vi "file -- scan filename logic -- V1.vi"(7 "scan fileneme action":T1, 8 "scan filename IN":T2={"mmddyy (str)"="", "counter (str)"="", "to F (kHz)"=0.0, "from F (kHz)"=0.0, "temperature (K)"=0.0, "date/time string"="", "time stamp"=timestamp(19856294.882018566 s since 1904-01-01), "base name"="", "temperature (str)"="", "from F (str)"="", "to F (str)"="", "format"=enum."no date string", "power (V)"=0.0, "power (str) "="", "Magn Field (T)"=0.0, "Magn Field (str)"=""}, 11 "base name IN":string="1.02000K_12_177_1.4V_Nov09-2012__12-14-10_001_110912") -> (0 "scan filename OUT":T2={"mmddyy (str)"="", "counter (str)"="", "to F (kHz)"=0.0, "from F (kHz)"=0.0, "temperature (K)"=0.0, "date/time string"="", "time stamp"=timestamp(19856294.882018566 s since 1904-01-01), "base name"="", "temperature (str)"="", "from F (str)"="", "to F (str)"="", "format"=enum."no date string", "power (V)"=0.0, "power (str) "="", "Magn Field (T)"=0.0, "Magn Field (str)"=""}, 1 "exact match":bool, 3 "string OUT":string)   [LabVIEW 2016]
uses:
  resonant_ultrasound/maglab ultrasound -- arkady/file -- scan filename.ctl
  resonant_ultrasound/maglab ultrasound -- arkady/file -- scan filename action.ctl
  <vilib>/regexp/Match Regular Expression.xnode
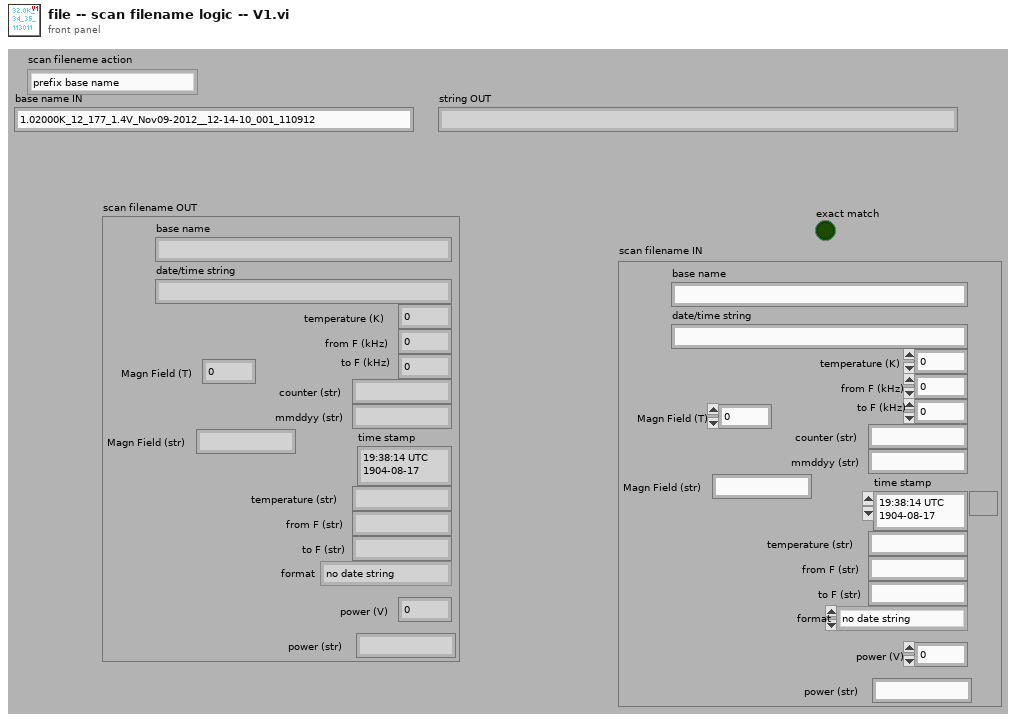
[diagram p1: front panel]
types:
  T1 = typedef "file -- scan filename action.ctl" = enum16{"prefix base name", "datestring regexp", "parse datestring", "datestring", "filename regexp", "parse filename", "datestring regexp (no brackets)", "suffix base name"}
  T2 = typedef "file -- scan filename.ctl" = cluster{"mmddyy (str)":string, "counter (str)":string, "to F (kHz)":dbl, "from F (kHz)":dbl, "temperature (K)":dbl, "date/time string":string, "time stamp":timestamp, "base name":string, "temperature (str)":string, "from F (str)":string, "to F (str)":string, "format":enum16{"no date string", "with date string"}, "power (V)":dbl, "power (str) ":string, "Magn Field (T)":dbl, "Magn Field (str)":string}
  T3 = typedef "LVDateTimeRec.ctl" = cluster{"fractional second":dbl, "second":i32, "minute":i32, "hour":i32, "day of month":i32, "month":i32, "year":i32, "day of week":i32, "day of year":i32, "DST":i32}
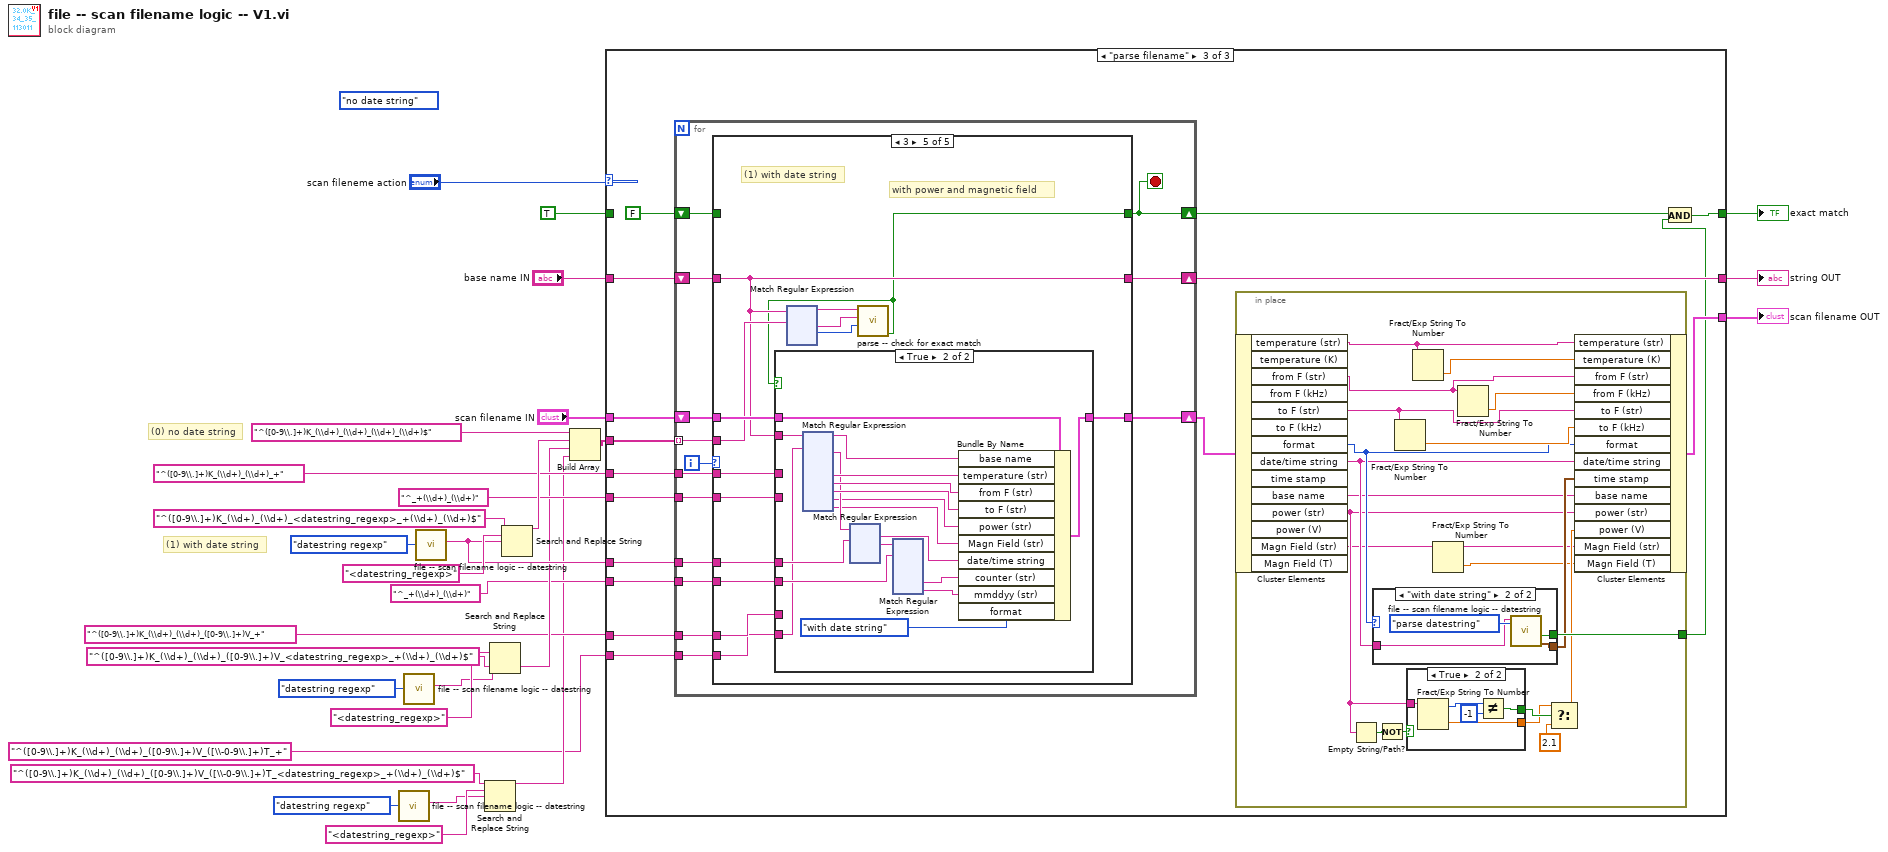
[diagram p0: block diagram]
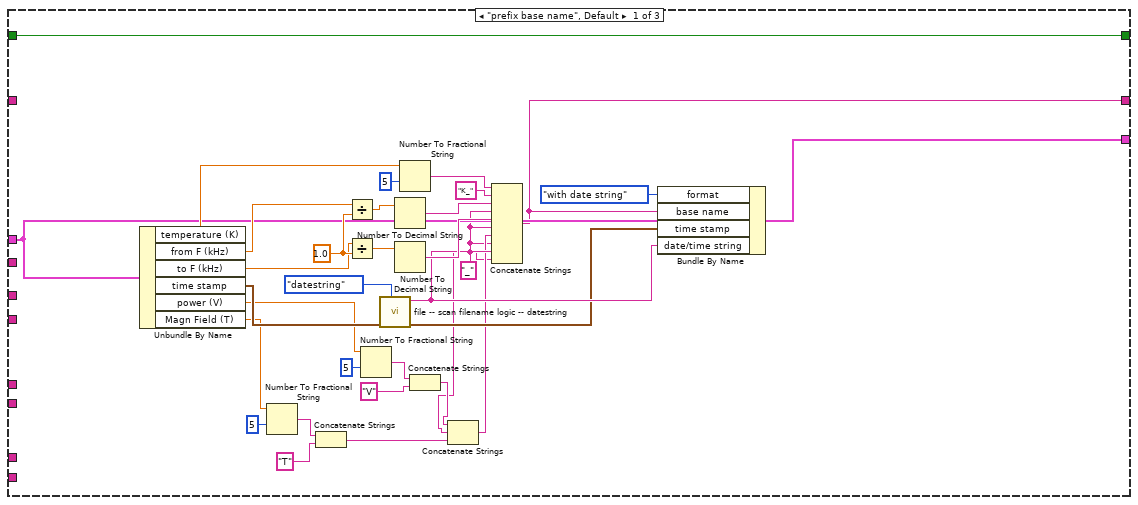
[diagram p2: hidden frame]
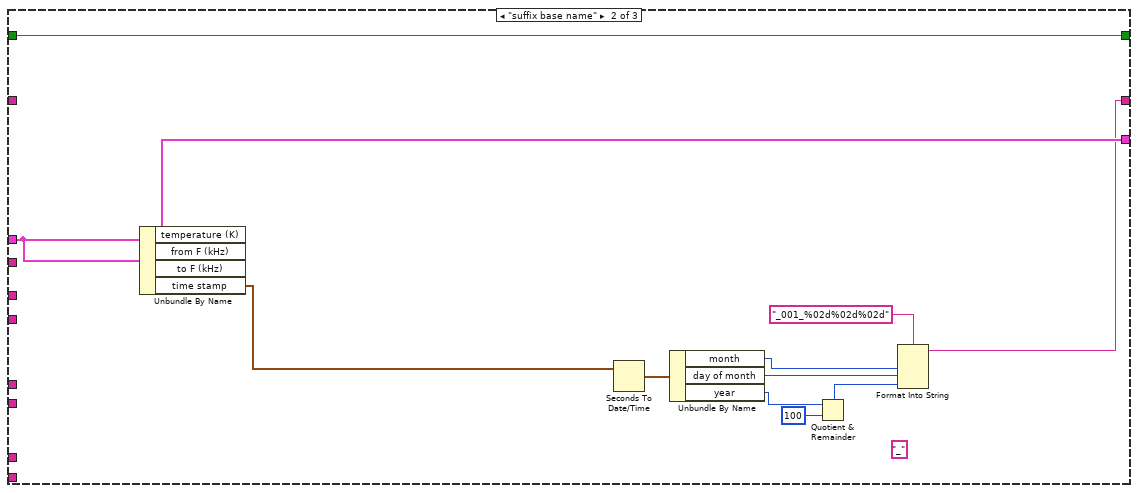
[diagram p3: hidden frame]
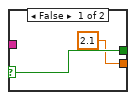
[diagram p4: hidden frame]
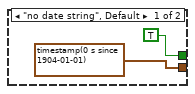
[diagram p5: hidden frame]
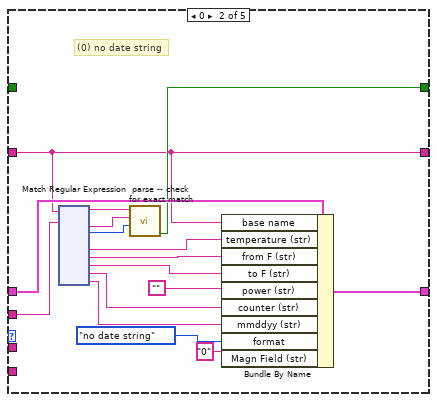
[diagram p7: hidden frame]
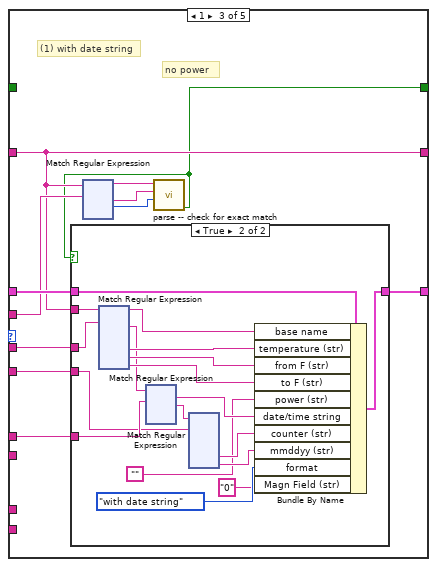
[diagram p8: hidden frame]
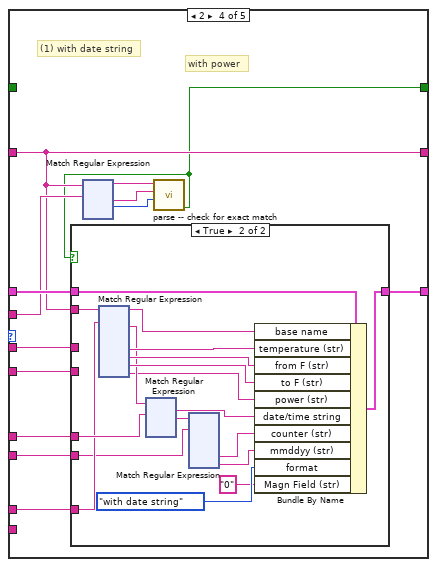
[diagram p10: hidden frame]
diagram:
  (unwired) enum16{"no date string", "with date string"}."no date string"
  # "(1) with date string"
  # "(0) no date string"
  n1 = call "file -- scan filename logic -- datestring.vi"("scan filename action"=file_--_scan_filename_action."datestring regexp") -> ("date string regexp"=w4:string)  [unwired: 7 in, 3 out]
  n2 = call "file -- scan filename logic -- datestring.vi"("scan filename action"=file_--_scan_filename_action."datestring regexp") -> ("date string regexp"=w11:string)  [unwired: 7 in, 3 out]
  n3 = call "file -- scan filename logic -- datestring.vi"("scan filename action"=file_--_scan_filename_action."datestring regexp") -> ("date string regexp"=w15:string)  [unwired: 7 in, 3 out]
  n4 = Search and Replace String(input string="^([0-9\\.]+)K_(\\d+)_(\\d+)_([0-9\\.]+)V_([\\-0-9\\.]+)T_<datestring_regexp>_+(\\d+)_(\\d+)$" ("string"), search string="<datestring_regexp>" ("string"), replace string=w4) -> (result string=w2:string)  [unwired: 5 in, 3 out]
  n5 = Search and Replace String(input string="^([0-9\\.]+)K_(\\d+)_(\\d+)_([0-9\\.]+)V_<datestring_regexp>_+(\\d+)_(\\d+)$" ("string"), search string="<datestring_regexp>" ("string"), replace string=w11) -> (result string=w9:string)  [unwired: 5 in, 3 out]
  n6 = Search and Replace String(input string="^([0-9\\.]+)K_(\\d+)_(\\d+)_<datestring_regexp>_+(\\d+)_(\\d+)$" ("string"), search string="<datestring_regexp>" ("string"), replace string=w15) -> (result string=w19:string)  [unwired: 5 in, 3 out]
  n7 = Build Array("^([0-9\\.]+)K_(\\d+)_(\\d+)_(\\d+)_(\\d+)$" ("string"), w19, w9, w2) -> (w18:string[])
  n8 = case shown="\"parse filename\"" "scan fileneme action" {
    tunnel: [w48 w72 w80] -> w29
    tunnel: "base name IN" -> [_ _ w84]
    tunnel: [w46 w67 w82] -> w17
    tunnel: "scan filename IN" -> [w47 w67 w88]
    tunnel: [w43 w62 w85] -> w25
    tunnel: TRUE -> [w48 w72 _]
    tunnel: w18 -> [_ _ w86]
    tunnel: "^([0-9\\.]+)K_(\\d+)_(\\d+)_+" ("string") -> [_ _ w78]
    tunnel: w15 -> [_ _ w77]
    tunnel: "^_+(\\d+)_(\\d+)" ("string") -> [_ _ w76]
    tunnel: "^([0-9\\.]+)K_(\\d+)_(\\d+)_([0-9\\.]+)V_+" ("string") -> [_ _ w75]
    tunnel: "^_+(\\d+)_(\\d+)" ("string") -> [_ _ w74]
    tunnel: "^([0-9\\.]+)K_(\\d+)_(\\d+)_([0-9\\.]+)V_([\\-0-9\\.]+)T_+" ("string") -> [_ _ w73]
    frame "prefix base name", Default {
      w57 = 1.0 ("y")
      w31 = "_" ("string")
      n9 = Unbundle By Name(w47) -> ("temperature (K)"=w50:dbl, "from F (kHz)"=w55:dbl, "to F (kHz)"=w56:dbl, "time stamp"=w49:timestamp, "power (V)"=w40:dbl, "Magn Field (T)"=w34:dbl)
      n10 = Number To Fractional String(number=w34, precision (6)=i16 5 ("width (-)")) -> (F-format string=w36:string)  [unwired: 2 in]
      n11 = Concatenate Strings(w36, "T" ("string")) -> (w30:string)
      n12 = Divide(x=w55, y=w57) -> (x/y=w60:dbl)
      n13 = Divide(x=w56, y=w57) -> (x/y=w59:dbl)
      n14 = Number To Fractional String(number=w40, precision (6)=i16 5 ("width (-)")) -> (F-format string=w39:string)  [unwired: 2 in]
      n15 = call "file -- scan filename logic -- datestring.vi"("scan filename action"=file_--_scan_filename_action."datestring", "time stamp IN"=w49) -> ("time stamp OUT"=w44:timestamp, "date/time string OUT"=w45:string)  [unwired: 6 in, 2 out]
      n16 = Number To Decimal String(number=w60) -> (decimal integer string=w51:string)  [unwired: 1 in]
      n17 = Number To Decimal String(number=w59) -> (decimal integer string=w52:string)  [unwired: 1 in]
      n18 = Number To Fractional String(number=w50, precision (6)=i16 5 ("width (-)")) -> (F-format string=w58:string)  [unwired: 2 in]
      n19 = Concatenate Strings(w39, "V" ("string")) -> (w33:string)
      n20 = Concatenate Strings(w33, w31, w30) -> (w32:string)
      n21 = Concatenate Strings(w58, "K_" ("string"), w51, w31, w52, w31, w32, w31, w45, w31) -> (w43:string)
      n22 = Bundle By Name(cluster=w47, "format"=enum16{"no date string", "with date string"}."with date string", "base name"=w43, "time stamp"=w44, "date/time string"=w45) -> (w46:T2)
    }
    frame "suffix base name" {
      (unwired) "_" ("string")
      n23 = Unbundle By Name(w67) -> ("time stamp"=w71:timestamp)  [unwired: 3 out]
      n24 = Seconds To Date/Time(time stamp (now)=w71) -> (date time rec=w70:T3)  [unwired: 1 in]
      n25 = Unbundle By Name(w70) -> ("month"=w66:i32, "day of month"=w65:i32, "year"=w69:i32)
      n26 = Quotient & Remainder(x=w69, y=100) -> (x-y*floor(x/y)=w64:i32)  [unwired: 1 out]
      n27 = Format Into String(format string="_001_%02d%02d%02d", w66, w65, w64) -> (resulting string=w62:string)  [unwired: 2 in, 1 out]
    }
    frame "parse filename" {
      n28 = for {
        shift-right: [w130] -> w81
        shift-left: FALSE -> [w128]
        tunnel: w86 -> [w133] mode=indexing
        shift-right: [w132] -> w85
        shift-left: w84 -> [w131]
        shift-right: [w129] -> w83
        shift-left: w88 -> [w135]
        tunnel: w78 -> [w127]
        tunnel: w77 -> [w126]
        tunnel: w76 -> [w125]
        tunnel: w75 -> [w124]
        tunnel: w74 -> [w123]
        tunnel: w73 -> [w122]
        i -> [w134]
        stop <- w130 stop-if-true
        n29 = case shown="3" w134 {
          tunnel: [w136 w153 w282 w764 w1248] -> w129
          tunnel: w135 -> [w136 w152 w281 w763 w1247]
          tunnel: w131 -> [w138 w146 w276 w758 w1242]
          tunnel: [w137 w148 w275 w757 w1241] -> w130
          tunnel: w133 -> [_ w147 w277 w759 w1243]
          tunnel: [w138 w146 w276 w758 w1242] -> w132
          tunnel: w128 -> [w137 _ _ _ _]
          tunnel: w127 -> [_ _ w274 w756 w1240]
          tunnel: w126 -> [_ _ w273 w755 w1239]
          tunnel: w125 -> [_ _ w272 w754 w1238]
          tunnel: w124 -> [_ _ _ w753 w1237]
          tunnel: w123 -> [_ _ _ w752 w1236]
          tunnel: w122 -> [_ _ _ _ w1235]
          frame -1, Default {
          }
          frame 0 {
            # "(0) no date string"
            n30 = xnode "Match Regular Expression"("input string"=w146, "regular expression"=w147) -> ("before match"=w151:string, "after match"=w150:string, "offset past match"=w149:i32, "submatch 1"=w142:string, "submatch 2"=w143:string, "submatch 3"=w144:string, "submatch 4"=w154:string, "submatch 5"=w145:string)  [unwired: 4 in, 2 out]
            n31 = call "parse -- check for exact match.vi"("offset past match"=w149, "after match"=w150, "before match"=w151) -> ("exact match"=w148:bool)  [unwired: 8 in]
            n32 = Bundle By Name(cluster=w152, "base name"=w146, "temperature (str)"=w142, "from F (str)"=w143, "to F (str)"=w144, "power (str)"="", "counter (str)"=w154, "mmddyy (str)"=w145, "format"=enum16{"no date string", "with date string"}."no date string", "Magn Field (str)"="0") -> (w153:T2)
          }
          frame 1 {
            # "no power"
            # "(1) with date string"
            n33 = xnode "Match Regular Expression"("input string"=w276, "regular expression"=w277) -> ("before match"=w280:string, "after match"=w279:string, "offset past match"=w278:i32)  [unwired: 4 in, 2 out]
            n34 = call "parse -- check for exact match.vi"("offset past match"=w278, "after match"=w279, "before match"=w280) -> ("exact match"=w275:bool)  [unwired: 8 in]
            n35 = case shown="True" w275 {
              tunnel: [w283 w300] -> w282
              tunnel: w281 -> [w283 w299]
              tunnel: w276 -> [_ w298]
              tunnel: w274 -> [_ w297]
              tunnel: w273 -> [_ w292]
              tunnel: w272 -> [_ w289]
              frame False {
              }
              frame True {
                n36 = xnode "Match Regular Expression"("input string"=w298, "regular expression"=w297) -> ("after match"=w293:string, "submatch 1"=w296:string, "submatch 2"=w295:string, "submatch 3"=w294:string)  [unwired: 4 in, 4 out]
                n37 = xnode "Match Regular Expression"("input string"=w293, "regular expression"=w292) -> ("whole match"=w291:string, "after match"=w290:string)  [unwired: 4 in, 3 out]
                n38 = xnode "Match Regular Expression"("input string"=w290, "regular expression"=w289) -> ("submatch 1"=w288:string, "submatch 2"=w287:string)  [unwired: 4 in, 5 out]
                n39 = Bundle By Name(cluster=w299, "base name"=w298, "temperature (str)"=w296, "from F (str)"=w295, "to F (str)"=w294, "power (str)"="", "date/time string"=w291, "counter (str)"=w288, "mmddyy (str)"=w287, "format"=enum16{"no date string", "with date string"}."with date string", "Magn Field (str)"="0") -> (w300:T2)
              }
            }
          }
          frame 2 {
            # "with power"
            # "(1) with date string"
            n40 = xnode "Match Regular Expression"("input string"=w758, "regular expression"=w759) -> ("before match"=w762:string, "after match"=w761:string, "offset past match"=w760:i32)  [unwired: 4 in, 2 out]
            n41 = call "parse -- check for exact match.vi"("offset past match"=w760, "after match"=w761, "before match"=w762) -> ("exact match"=w757:bool)  [unwired: 8 in]
            n42 = case shown="True" w757 {
              tunnel: [w765 w782] -> w764
              tunnel: w763 -> [w765 w781]
              tunnel: w758 -> [_ w780]
              tunnel: w756 -> [_ _]
              tunnel: w755 -> [_ w775]
              tunnel: w754 -> [_ _]
              tunnel: w753 -> [_ w768]
              tunnel: w752 -> [_ w767]
              frame False {
              }
              frame True {
                n43 = xnode "Match Regular Expression"("input string"=w780, "regular expression"=w768) -> ("after match"=w776:string, "submatch 1"=w779:string, "submatch 2"=w778:string, "submatch 3"=w777:string, "submatch 4"=w769:string)  [unwired: 4 in, 4 out]
                n44 = xnode "Match Regular Expression"("input string"=w776, "regular expression"=w775) -> ("whole match"=w774:string, "after match"=w773:string)  [unwired: 4 in, 3 out]
                n45 = xnode "Match Regular Expression"("input string"=w773, "regular expression"=w767) -> ("submatch 1"=w772:string, "submatch 2"=w771:string)  [unwired: 4 in, 5 out]
                n46 = Bundle By Name(cluster=w781, "base name"=w780, "temperature (str)"=w779, "from F (str)"=w778, "to F (str)"=w777, "power (str)"=w769, "date/time string"=w774, "counter (str)"=w772, "mmddyy (str)"=w771, "format"=enum16{"no date string", "with date string"}."with date string", "Magn Field (str)"="0") -> (w782:T2)
              }
            }
          }
          frame 3 {
            # "with power and magnetic field"
            # "(1) with date string"
            n47 = xnode "Match Regular Expression"("input string"=w1242, "regular expression"=w1243) -> ("before match"=w1246:string, "after match"=w1245:string, "offset past match"=w1244:i32)  [unwired: 4 in, 2 out]
            n48 = call "parse -- check for exact match.vi"("offset past match"=w1244, "after match"=w1245, "before match"=w1246) -> ("exact match"=w1241:bool)  [unwired: 8 in]
            n49 = case shown="True" w1241 {
              tunnel: [w1249 w1266] -> w1248
              tunnel: w1247 -> [w1249 w1265]
              tunnel: w1242 -> [_ w1264]
              tunnel: w1240 -> [_ _]
              tunnel: w1239 -> [_ w1259]
              tunnel: w1238 -> [_ _]
              tunnel: w1237 -> [_ _]
              tunnel: w1236 -> [_ w1252]
              tunnel: w1235 -> [_ w1251]
              frame False {
              }
              frame True {
                n50 = xnode "Match Regular Expression"("input string"=w1264, "regular expression"=w1251) -> ("after match"=w1260:string, "submatch 1"=w1263:string, "submatch 2"=w1262:string, "submatch 3"=w1261:string, "submatch 4"=w1253:string, "submatch 5"=w1250:string)  [unwired: 4 in, 4 out]
                n51 = xnode "Match Regular Expression"("input string"=w1260, "regular expression"=w1259) -> ("whole match"=w1258:string, "after match"=w1257:string)  [unwired: 4 in, 3 out]
                n52 = xnode "Match Regular Expression"("input string"=w1257, "regular expression"=w1252) -> ("submatch 1"=w1256:string, "submatch 2"=w1255:string)  [unwired: 4 in, 5 out]
                n53 = Bundle By Name(cluster=w1265, "base name"=w1264, "temperature (str)"=w1263, "from F (str)"=w1262, "to F (str)"=w1261, "power (str)"=w1253, "Magn Field (str)"=w1250, "date/time string"=w1258, "counter (str)"=w1256, "mmddyy (str)"=w1255, "format"=enum16{"no date string", "with date string"}."with date string") -> (w1266:T2)
              }
            }
          }
        }
      }
      n54 = in-place {
        in-place-border: [w100] -> w79
        n55 = in-place-cluster #1(w83) -> ("temperature (str)"=w107:string, "from F (str)"=w106:string, "to F (str)"=w104:string, "format"=w102:enum16{"no date string", "with date string"}, "date/time string"=w101:string, "base name"=w98:string, "power (str)"=w91:string, "Magn Field (str)"=w90:string)  [unwired: 6 out]
        n56 = Empty String/Path?(string/path=w91) -> (empty?=w97:bool)
        n57 = case shown="\"with date string\"" w102 {
          tunnel: w101 -> [_ w120]
          tunnel: [TRUE w119] -> w100
          tunnel: [timestamp(0 s since 1904-01-01) ("time stamp OUT") w118] -> w99
          frame "no date string", Default {
          }
          frame "with date string" {
            n58 = call "file -- scan filename logic -- datestring.vi"("scan filename action"=file_--_scan_filename_action."parse datestring", "date/time string IN"=w120) -> ("time stamp OUT"=w118:timestamp, "parse OK"=w119:bool)  [unwired: 6 in, 2 out]
          }
        }
        n59 = Not(x=w97) -> (.not. x?=w96:bool)
        n60 = Fract/Exp String To Number(string=w104) -> (number=w103:dbl)  [unwired: 3 in, 1 out]
        n61 = case shown="True" w96 {
          selector: w96 -> [w110 _]
          tunnel: [w110 w112] -> w95
          tunnel: w91 -> [_ w115]
          tunnel: [2.1 w111] -> w93
          frame False {
          }
          frame True {
            n62 = Fract/Exp String To Number(string=w115) -> (offset past number=w114:i32, number=w111:dbl)  [unwired: 3 in]
            n63 = Not Equal?(x=w114, y=-1) -> (x != y?=w112:bool)
          }
        }
        n64 = Fract/Exp String To Number(string=w107) -> (number=w108:dbl)  [unwired: 3 in, 1 out]
        n65 = Fract/Exp String To Number(string=w90) -> (number=w89:dbl)  [unwired: 3 in, 1 out]
        n66 = Fract/Exp String To Number(string=w106) -> (number=w105:dbl)  [unwired: 3 in, 1 out]
        n67 = Select(t=w93, s=w95, f=2.1) -> (s? t:f=w92:dbl)
        n68 = in-place-cluster #1("temperature (str)"=w107, "temperature (K)"=w108, "from F (str)"=w106, "from F (kHz)"=w105, "to F (str)"=w104, "to F (kHz)"=w103, "format"=w102, "date/time string"=w101, "time stamp"=w99, "base name"=w98, "power (str)"=w91, "power (V)"=w92, "Magn Field (str)"=w90, "Magn Field (T)"=w89) -> (w82:T2)
      }
      n69 = And(x=w81, y=w79) -> (x .and. y?=w80:bool)
    }
  }
  "exact match" <- w29
  "scan filename OUT" <- w17
  "string OUT" <- w25
